vi "CPU_P_get_flag.vi"(7 "flag":enum8{"C", "Z", "I", "D", "B", "V", "N"}(ring), 11 "registers":T1={"A"=0, "X"=0, "Y"=0, "SP"=253, "PC"=0, "P"=36} {"P" format="%08b"; "PC" format="%04x"; "SP" format="%02x"; "Y" format="%02x"; "X" format="%02x"; "A" format="%02x"}) -> (2 "Value":bool, 3 "registers":T1={"A"=0, "X"=0, "Y"=0, "SP"=253, "PC"=0, "P"=36} {"P" format="%08b"; "PC" format="%04x"; "SP" format="%02x"; "Y" format="%02x"; "X" format="%02x"; "A" format="%02x"})   [LabVIEW 2018]
uses:
  CPU_registers.ctl
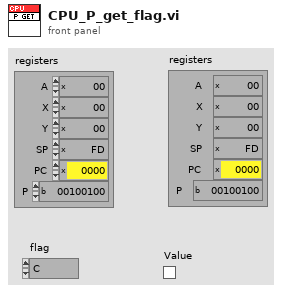
[diagram p1: front panel]
types:
  T1 = typedef "CPU_registers.ctl" = cluster{"A":u8, "X":u8, "Y":u8, "SP":u8, "PC":u16, "P":u8}
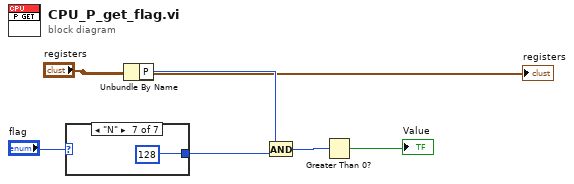
[diagram p0: block diagram]
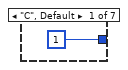
[diagram p2: hidden frame]
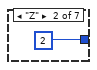
[diagram p3: hidden frame]
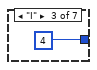
[diagram p4: hidden frame]
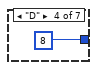
[diagram p5: hidden frame]
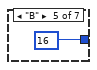
[diagram p6: hidden frame]
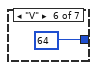
[diagram p7: hidden frame]
diagram:
  n1 = case shown="\"N\"" "flag" {
    tunnel: [u8 1 u8 2 u8 4 u8 8 u8 16 u8 64 u8 128] -> w3
    frame "C", Default {
    }
    frame "Z" {
    }
    frame "I" {
    }
    frame "D" {
    }
    frame "B" {
    }
    frame "V" {
    }
    frame "N" {
    }
  }
  n2 = Unbundle By Name("registers") -> ("P"=w5:u8)
  n3 = And(x=w5, y=w3) -> (x .and. y?=w2:u8)
  n4 = Greater Than 0?(x=w2) -> (x > 0?=→"Value":bool)
  "registers" <- "registers"
